vi "Map.vi"(7 "Action":enum8{"noop", "get", "set", "pop"}(ring), 10 "Queue in":refnum<queue>, 11 "Queue Name":string) -> (1 "Found?":bool, 2 "Queue out":refnum<queue>, 3 "Queue Map":map{string, refnum<queue>}(c390))   [LabVIEW 2021, in "Queue.lvlib"]
uses:
  Queue.lvlib
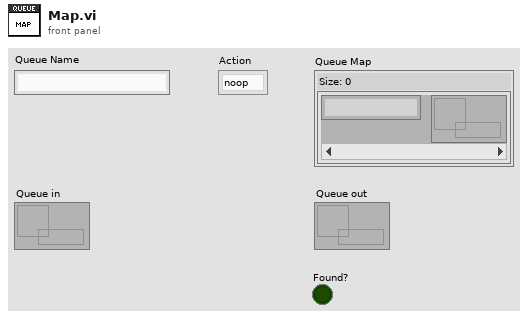
[diagram p1: front panel]
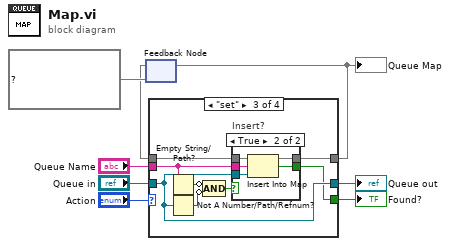
[diagram p0: block diagram]
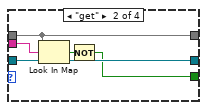
[diagram p3: hidden frame]
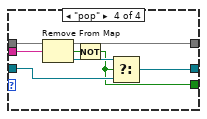
[diagram p5: hidden frame]
diagram:
  n1 = feedback #1(map{string, refnum<queue>} {} ("Queues")) -> (w5:map{string, refnum<queue>})
  n2 = case shown="\"set\"" "Action" {
    tunnel: [w9 w13 w19 w32] -> w8
    tunnel: "Queue Name" -> [_ w14 w24 w36]
    tunnel: w5 -> [w10 w16 w23 w38]
    tunnel: [w10 w16 w22 w37] -> w4
    tunnel: [_ w11 w17 w31] -> w3
    tunnel: "Queue in" -> [w9 w15 w19 w34]
    frame "noop" {
    }
    frame "get" {
      n3 = Look In Map(map=w16, key=w14, default value=w15) -> (key not found?=w12:bool, value=w13:refnum<queue>)
      n4 = Not(x=w12) -> (.not. x?=w11:bool)
    }
    frame "set" {
      n5 = Empty String/Path?(string/path=w24) -> (empty?=w21:bool)
      n6 = Not A Number/Path/Refnum?(number/path/refnum=w19) -> (NaN/Path/Refnum?=w18:bool)
      n7 = Compound Arithmetic op=AND(invert w21, invert w18) -> (w20:bool)
      n8 = case "Insert?" shown="True" w20 {
        tunnel: w23 -> [w25 w30]
        tunnel: w19 -> [_ w29]
        tunnel: w24 -> [_ w28]
        tunnel: [w25 w27] -> w22
        tunnel: [_ w26] -> w17
        frame False {
        }
        frame True {
          n9 = Insert Into Map(map in=w30, key=w28, value=w29) -> (map out=w27:map{string, refnum<queue>}, key already included?=w26:bool)  [unwired: 1 out]
        }
      }
    }
    frame "pop" {
      n10 = Remove From Map(10:w36, 11:w38) -> (1:w33:refnum<queue>, 2:w35:bool, 3:w37:map{string, refnum<queue>})
      n11 = Not(x=w35) -> (.not. x?=w31:bool)
      n12 = Select(t=w33, s=w31, f=w34) -> (s? t:f=w32:refnum<queue>)
    }
  }
  "Queue out" <- w8
  "Found?" <- w3
  "Queue Map" <- w4
  n13 = feedback-in #1(w4) -> ()
